vi "USRP Packet Transmitter(working).vi"(8 "Tx Parameters":T7={"Tx IQ Sampling\nRate [s/sec]"=500000.0, "Tx Frequency [Hz]"=2500000000.0, "Tx Gain [dB]"=0.0, "Tx Antenna"="TX1"} {"Tx Gain [dB]" format="%#.6p"; "Tx Frequency [Hz]" format="%#.6p"; "Tx IQ Sampling\nRate [s/sec]" format="%#.6p"}, 9 "USRP IP address":refnum<k15>="192.168.10.2", 10 "working directory":path=path "C:/perlTest") -> (1 "Constellation Graph":T1(graph), 2 "error out":errorcluster, 3 "standard output":string)   [LabVIEW 2022 SP3]
uses:
  <instrlib>/niUSRP/niUSRP Write Tx Data (CDB Cluster).vi
  <vilib>/addons/Modulation/Digital/General/MT Generate PSK System Parameters(M).vi
  <vilib>/addons/Modulation/niDMT.lvlib
panel:
  out "error out 2":errorcluster
  in  "autoscale":bool
  out "Symbol Rate\n[symbols/sec]":dbl=25000.0 format="%#.6p"
  in  "stop":bool
  in  "Tab Control":T2(tab)
  in  "command line":string
  in  "Packet Parameters":T3={"Guard Bits "=30, "Sync Bits"=20, "Message Bits"=128}
  in  "Packet Pad \n[samples]":i32=200
  in  "Blank Frame \n[samples]":i32=500
  out "Number of Packets in Message":i32=46
  in  "PN sequence order\nfor Sync Bits":i32=31 caption="PN sequence order (9)"
  in  "Packet Repeat":i32=2
  in  "Select PSK Modulation Format":T4(tab)=enum."QPSK" caption="PSK"
  in  "BPSK System Parameters":T5={"Samples per Symbol"=8, "symbol map"=[], "Differential PSK"=enum."disable", "PSK type"=0} {"PSK type" items=["normal", "shifted", "offset"]; "symbol map" format="%.3f"}
  in  "QPSK System Parameters":T5={"Samples per Symbol"=8, "symbol map"=[], "Differential PSK"=enum."disable", "PSK type"=0} {"PSK type" items=["normal", "shifted", "offset"]; "symbol map" format="%.3f"}
  in  "pi/4 DQPSK System Parameters":T5={"Samples per Symbol"=8, "symbol map"=[], "Differential PSK"=enum."enable", "PSK type"=1} {"PSK type" items=["normal", "shifted", "offset"]; "symbol map" format="%.3f"}
  in  "OQPSK System Parameters":T5={"Samples per Symbol"=8, "symbol map"=[], "Differential PSK"=enum."disable", "PSK type"=2} {"PSK type" items=["normal", "shifted", "offset"]; "symbol map" format="%.3f"}
  in  "8-PSK System Parameters":T5={"Samples per Symbol"=8, "symbol map"=[], "Differential PSK"=enum."disable", "PSK type"=0} {"PSK type" items=["normal", "shifted", "offset"]; "symbol map" format="%.3f"}
  in  "16-PSK System Parameters":T5={"Samples per Symbol"=8, "symbol map"=[], "Differential PSK"=enum."disable", "PSK type"=0} {"PSK type" items=["normal", "shifted", "offset"]; "symbol map" format="%.3f"}
  in  "M":i32=4 min=2 step=2
  in  "Custom System Parameters":T5={"Samples per Symbol"=8, "symbol map"=[], "Differential PSK"=enum."disable", "PSK type"=0} {"PSK type" items=["normal", "shifted", "offset"]; "symbol map" format="%.3f"}
  in  "Pulse Shaping Filter Parameters":T6={"Alpha"=0.5, "Filter Length"=6, "TX Filter"=enum."Root Raised Cos"} caption="Pulse Shaping Filter" {"Alpha" format="%.2f"}
  out "Actual Tx Parameters":T7={"Tx IQ Sampling\nRate [s/sec]"=200000.0, "Tx Frequency [Hz]"=2500000000.0, "Tx Gain [dB]"=0.0, "Tx Antenna"="TX1"} {"Tx Gain [dB]" format="%#.6p"; "Tx Frequency [Hz]" format="%#.6p"; "Tx IQ Sampling\nRate [s/sec]" format="%#.6p"}
  in  "Queue Length":i32=10
  # "Packet Transmitter"
  # "Guard\nBand"
  # "Sync\nSeq"
  # "Packet\nNumber"
  # "Pad\nData"
  # "Blank\nFrame"
  # "Data"
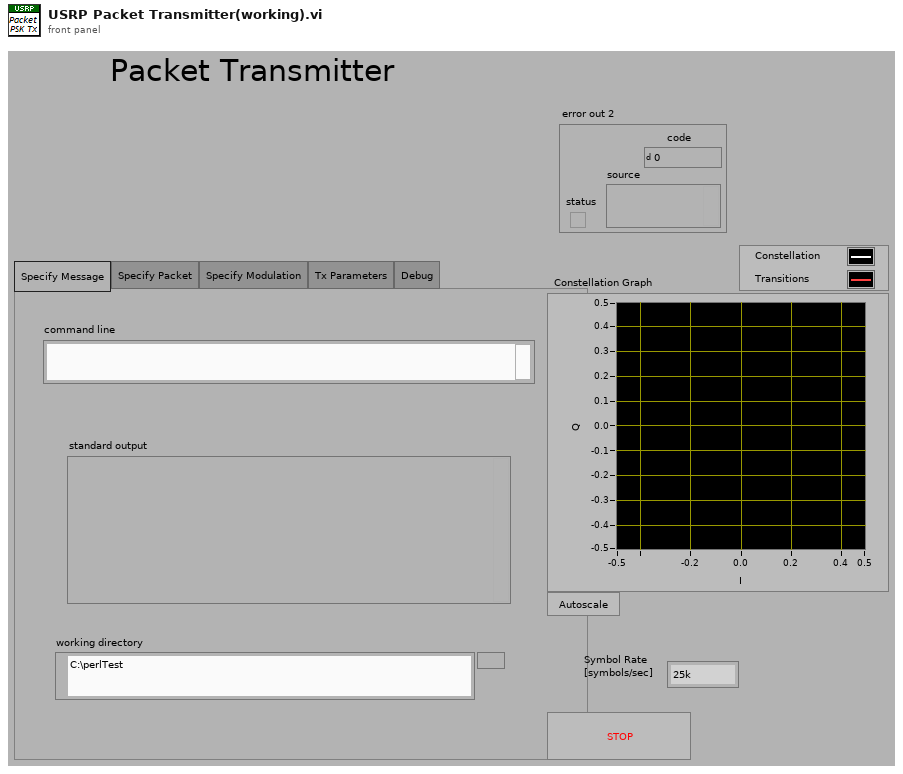
[diagram p1: front panel]
types:
  T1 = cluster{"Decimated Array":dbl[], "Decimated Array":dbl[]}[]
  T2 = enum32{"Specify Message", "Specify Packet", "Specify Modulation", "Tx Parameters", "Debug"}
  T3 = cluster{"Guard Bits ":i32, "Sync Bits":i32, "Message Bits":i32}
  T4 = enum32{"BPSK", "QPSK", "pi/4DQPSK", "OQPSK", "8-PSK", "16-PSK", "Custom"}
  T5 = cluster{"Samples per Symbol":i32, "symbol map":cdb[], "Differential PSK":enum16{"disable", "enable"}, "PSK type":u16}
  T6 = cluster{"Alpha":dbl, "Filter Length":i32, "TX Filter":enum16{"none", "Raised Cosine", "Root Raised Cos", "Gaussian"}}
  T7 = cluster{"Tx IQ Sampling\nRate [s/sec]":dbl, "Tx Frequency [Hz]":dbl, "Tx Gain [dB]":dbl, "Tx Antenna":string}
  T8 = cluster{"samples per symbol (16)":i32, "symbol map":cdb[], "differential PSK":enum16{"disable", "enable"}, "PSK type":u16}
  T9 = cluster{"s? t:f":cluster{"t0":dbl, "dt":dbl, "Y":cdb[]}, i32}
  T10 = cluster{"output complex waveform":cluster{"t0":dbl, "dt":dbl, "Y":cdb[]}, i32}
  T11 = cluster{"constellation":dbl[], "oversampled data":dbl[]}[]
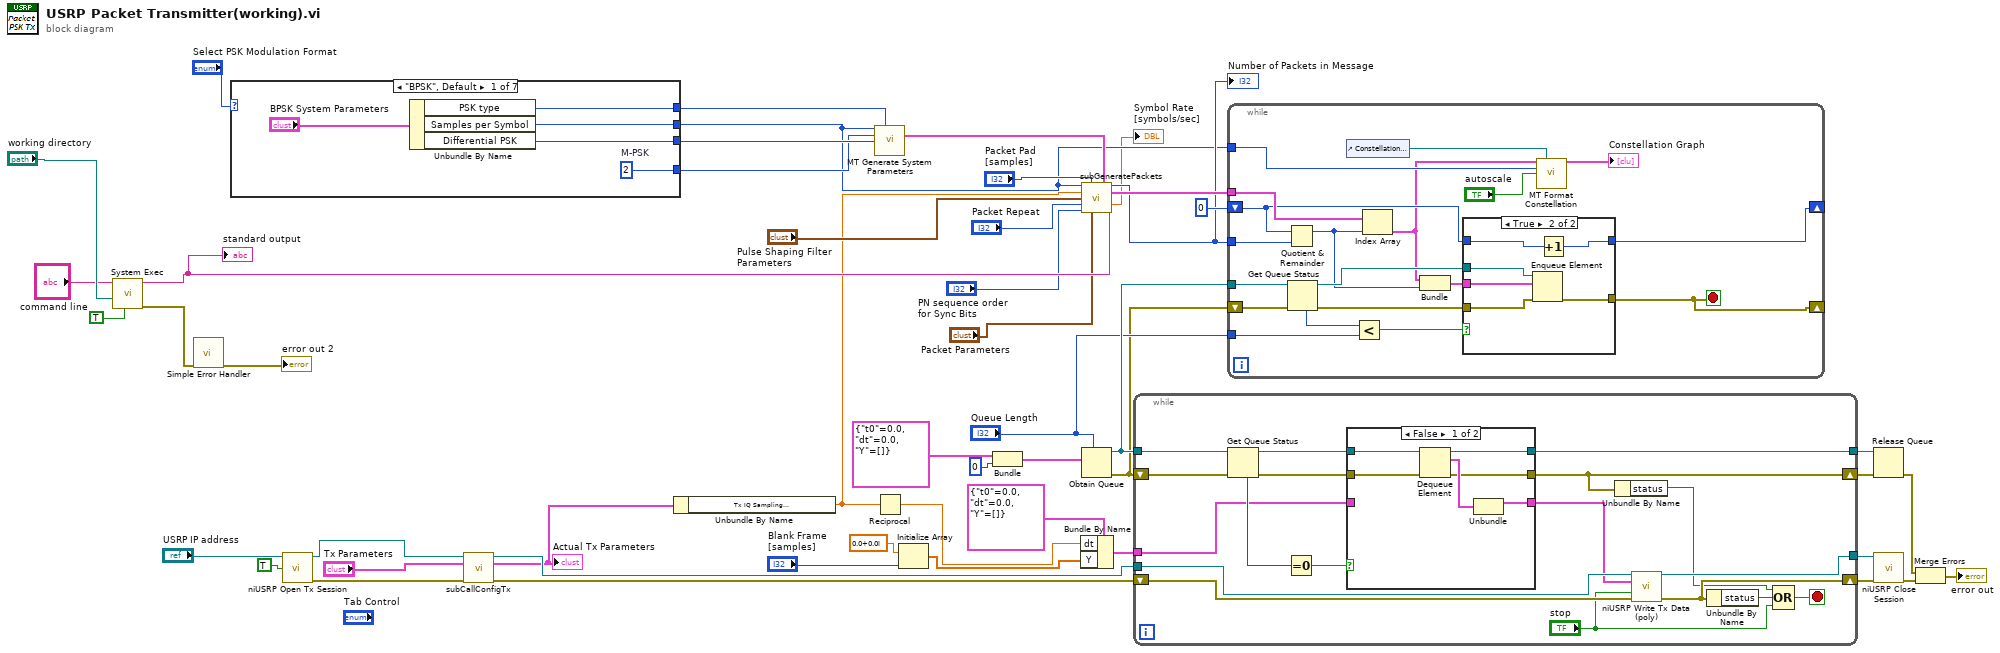
[diagram p0: block diagram]
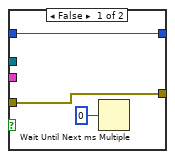
[diagram p2: hidden frame]
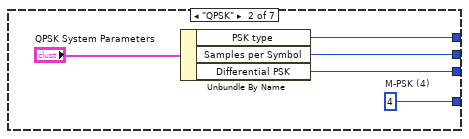
[diagram p3: hidden frame]
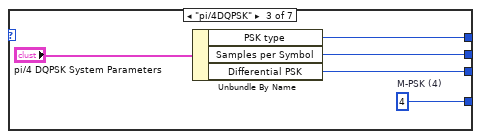
[diagram p4: hidden frame]
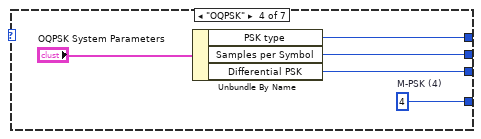
[diagram p5: hidden frame]
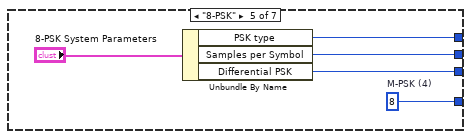
[diagram p6: hidden frame]
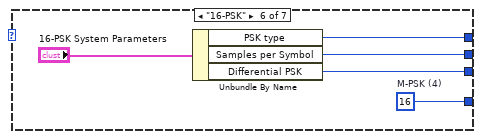
[diagram p7: hidden frame]
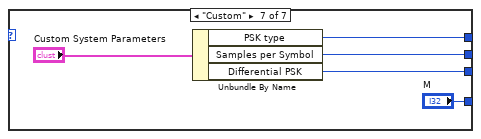
[diagram p8: hidden frame]
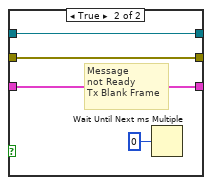
[diagram p9: hidden frame]
diagram:
  n1 = call <vilib>:"System Exec.vi"("run minimized? (F)"=TRUE, "working directory"="working directory", "command line"="command line") -> ("error out"=w3:errorcluster, "standard output"=w48:string)  [unwired: 3 in, 4 out]
  "standard output" <- w48
  n2 = call <vilib>:"Simple Error Handler.vi"("error in (no error)"=w3) -> ("error out"=→"error out 2":errorcluster)  [unwired: 1 in, 7 out]
  n3 = case shown="\"BPSK\", Default" "Select PSK Modulation Format" {
    tunnel: [w51 w55 w63 w68 w73 w79 w82] -> w7
    tunnel: [w52 w57 w62 w67 w72 w78 w83] -> w46
    tunnel: [w54 w59 w64 w69 w71 w77 "M"] -> w28
    tunnel: [w53 w58 w61 w66 w74 w76 w84] -> w15
    frame "BPSK", Default {
      w54 = 2  # M-PSK
      n4 = Unbundle By Name("BPSK System Parameters") -> ("PSK type"=w53:u16, "Samples per Symbol"=w51:i32, "Differential PSK"=w52:enum16{"disable", "enable"})
    }
    frame "QPSK" {
      w59 = 4  # M-PSK (4)
      n5 = Unbundle By Name("QPSK System Parameters") -> ("PSK type"=w58:u16, "Samples per Symbol"=w55:i32, "Differential PSK"=w57:enum16{"disable", "enable"})
    }
    frame "pi/4DQPSK" {
      w64 = 4  # M-PSK (4)
      n6 = Unbundle By Name("pi/4 DQPSK System Parameters") -> ("PSK type"=w61:u16, "Samples per Symbol"=w63:i32, "Differential PSK"=w62:enum16{"disable", "enable"})
    }
    frame "OQPSK" {
      w69 = 4  # M-PSK (4)
      n7 = Unbundle By Name("OQPSK System Parameters") -> ("PSK type"=w66:u16, "Samples per Symbol"=w68:i32, "Differential PSK"=w67:enum16{"disable", "enable"})
    }
    frame "8-PSK" {
      w71 = 8  # M-PSK (4)
      n8 = Unbundle By Name("8-PSK System Parameters") -> ("PSK type"=w74:u16, "Samples per Symbol"=w73:i32, "Differential PSK"=w72:enum16{"disable", "enable"})
    }
    frame "16-PSK" {
      w77 = 16  # M-PSK (4)
      n9 = Unbundle By Name("16-PSK System Parameters") -> ("PSK type"=w76:u16, "Samples per Symbol"=w79:i32, "Differential PSK"=w78:enum16{"disable", "enable"})
    }
    frame "Custom" {
      n10 = Unbundle By Name("Custom System Parameters") -> ("PSK type"=w84:u16, "Samples per Symbol"=w82:i32, "Differential PSK"=w83:enum16{"disable", "enable"})
    }
  }
  n11 = call <instrlib>:"niUSRP Open Tx Session.vi"("device names"="USRP IP address", "reset"=TRUE) -> ("session handle out"=w19:refnum<k15>, "error out"=w18:errorcluster)  [unwired: 12 in]
  n12 = call "subCallConfigTx.vi"("session handle"=w19, "Tx Parameters"="Tx Parameters", "error in"=w18) -> ("session handle out"=w27:refnum<k15>, "Actual Tx Parameters"=w26:T7, "error out"=w32:errorcluster)  [unwired: 10 in]
  "Actual Tx Parameters" <- w26
  n13 = Unbundle By Name(w26) -> ("Tx IQ Sampling\nRate [s/sec]"=w8:dbl)
  n14 = call-poly <vilib>:"MT Generate System Parameters.vi"("samples per symbol (16)"=w7, "PSK type"=w15, "M-PSK (4)"=w28, "differential PSK"=w46) -> ("PSK system parameters"=w16:T8)  [unwired: 9 in, 2 out]
  n15 = Reciprocal(x=w8) -> (1/x=w29:dbl)
  n16 = Initialize Array(cdb 0.0+0.0i ("element"), "Blank Frame \n[samples]") -> (w42:cdb[])
  n17 = Bundle("s? t:f"=cluster{"t0":dbl, "dt":dbl, "Y":cdb[]} {"t0"=0.0, "dt"=0.0, "Y"=[]}, 0) -> (w37:T9)  [unwired: 1 in]
  n18 = Bundle By Name(cluster=cluster{"t0":dbl, "dt":dbl, "Y":cdb[]} {"t0"=0.0, "dt"=0.0, "Y"=[]} ("s? t:f"), "dt"=w29, "Y"=w42) -> (w41:cluster{"t0":dbl, "dt":dbl, "Y":cdb[]})
  n19 = call "subGeneratePackets.vi"("Samples per Symbol"=w7, "Packet Pad \n[samples]"="Packet Pad \n[samples]", "PSK system parameters"=w16, "Tx IQ Sampling\nRate [s/sec]"=w8, "Pulse Shaping Filter Parameters"="Pulse Shaping Filter Parameters", "Packet Repeat"="Packet Repeat", "PN sequence order\nfor Sync Bits"="PN sequence order\nfor Sync Bits", "Packet Parameters"="Packet Parameters", "Message Text"=w48) -> ("Number of Packets"=w25:i32, "Packets"=w34:cluster{"t0":dbl, "dt":dbl, "Y":cdb[]}[], "Symbol Rate"=→"Symbol Rate\n[symbols/sec]":dbl)  [unwired: 4 in]
  "Number of Packets in Message" <- w25
  n20 = Obtain Queue(max queue size (-1, unlimited)="Queue Length", element data type=w37) -> (queue out=w43:refnum<queue>, error out=w21:errorcluster)  [unwired: 3 in, 1 out]
  n21 = while {
    tunnel: w27 -> [w93]
    shift-right: [w90] -> w31
    shift-left: w32 -> [w94]
    tunnel: w43 -> [w102]
    tunnel: w41 -> [w99]
    tunnel: [w98] -> w40
    tunnel: [w92] -> w30
    shift-right: [w87] -> w39
    shift-left: w21 -> [w95]
    stop <- w89 stop-if-true
    n22 = Get Queue Status(queue=w102, error in (no error)=w95) -> (queue out=w97:refnum<queue>, error out=w96:errorcluster, # elements in queue=w101:i32)  [unwired: 1 in, 5 out]
    n23 = Equal To 0?(x=w101) -> (x = 0?=w100:bool)
    n24 = case shown="False" w100 {
      tunnel: w99 -> [_ w112]
      tunnel: [w104 w112] -> w85
      tunnel: [w108 w110] -> w98
      tunnel: [w103 w111] -> w87
      tunnel: w97 -> [w107 w110]
      tunnel: w96 -> [w106 w111]
      frame False {
        n25 = Dequeue Element(queue=w107, error in (no error)=w106) -> (queue out=w108:refnum<queue>, element=w105:T9, error out=w103:errorcluster)  [unwired: 1 in, 1 out]
        n26 = Unbundle(w105) -> ("s? t:f"=w104:cluster{"t0":dbl, "dt":dbl, "Y":cdb[]})  [unwired: 1 out]
      }
      frame True {
        # "Message\nnot Ready\nTx Blank Frame"
        n27 = Wait Until Next ms Multiple(millisecond multiple=u32 0) -> ()  [unwired: 1 out]
      }
    }
    n28 = Unbundle By Name(w87) -> ("status"=w86:bool)
    n29 = call-poly <instrlib>:"niUSRP Write Tx Data (poly).vi"("session handle"=w93, "data"=w85, "end of data?"="stop", "error in (no error)"=w94) -> ("session handle out"=w92:refnum<k15>, "error out"=w90:errorcluster)  [unwired: 10 in]
    n30 = Unbundle By Name(w90) -> ("status"=w91:bool)
    n31 = Compound Arithmetic op=OR(w86, w91, "stop") -> (w89:bool)
  }
  n32 = while {
    tunnel: w43 -> [w131]
    shift-right: [w124] -> _
    shift-left: 0 -> [w120]
    tunnel: w34 -> [w121]
    tunnel: "Queue Length" -> [w123]
    tunnel: w25 -> [w122]
    shift-right: [w118] -> _
    shift-left: w21 -> [w126]
    tunnel: w7 -> [w115]
    stop <- w118 stop-if-true
    n33 = Quotient & Remainder(x=w120, y=w122) -> (x-y*floor(x/y)=w119:i32)  [unwired: 1 out]
    n34 = Get Queue Status(queue=w131, error in (no error)=w126) -> (queue out=w130:refnum<queue>, error out=w127:errorcluster, # elements in queue=w129:i32)  [unwired: 1 in, 5 out]
    n35 = control-ref of="Constellation Graph"() -> (w116:refnum<vi>)
    n36 = Less?(x=w129, y=w123) -> (x < y?=w128:bool)
    n37 = Index Array(array=w121, index=w119) -> (element=w113:cluster{"t0":dbl, "dt":dbl, "Y":cdb[]})
    n38 = Bundle("output complex waveform"=w113, w119) -> (w125:T10)  [unwired: 1 in]
    n39 = case shown="True" w128 {
      tunnel: w127 -> [w132 w140]
      tunnel: w130 -> [_ w139]
      tunnel: [w132 w138] -> w118
      tunnel: w125 -> [_ w137]
      tunnel: w120 -> [w134 w136]
      tunnel: [w134 w135] -> w124
      frame False {
        n40 = Wait Until Next ms Multiple(millisecond multiple=u32 0) -> ()  [unwired: 1 out]
      }
      frame True {
        n41 = Enqueue Element(queue=w139, element=w137, error in (no error)=w140) -> (error out=w138:errorcluster)  [unwired: 1 in, 2 out]
        n42 = Increment(x=w136) -> (x+1=w135:i32)
      }
    }
    n43 = call <vilib>:"MT Format Constellation.vi"("waveform"=w113, "constellation reference"=w116, "samples per symbol"=w115, "autoscale"="autoscale") -> ("constellation graph"=→"Constellation Graph":T11)  [unwired: 1 in, 10 out]
  }
  n44 = Release Queue(queue=w40, error in (no error)=w39) -> (error out=w14:errorcluster)  [unwired: 3 out]
  n45 = call <instrlib>:"niUSRP Close Session.vi"("session handle"=w30, "error in (no error)"=w31) -> ("error out"=w13:errorcluster)  [unwired: 13 in]
  n46 = Merge Errors(w14, w13) -> (→"error out":errorcluster)
